vi "getDefaultData.vi"(8 "error in (no error)":errorcluster, 11 "DeviceData in":refnum<class "DeviceData.lvclass">) -> (0 "error out":errorcluster, 1 "calibratedValues":dbl[](array[numeric]), 2 "channelAddresses":string[](array[string]), 3 "DeviceData out":refnum<class "DeviceData.lvclass">)   [LabVIEW 2009, in "DataMappers.lvlib" / "DeviceData.lvclass"]
uses:
  DeviceData.lvclass
  DeviceData.lvclass/DeviceData.ctl
  DatabaseHelpers/Database Objects/ChannelArray/ChannelArray.lvclass
  DatabaseHelpers/Database Objects/device/device.lvclass
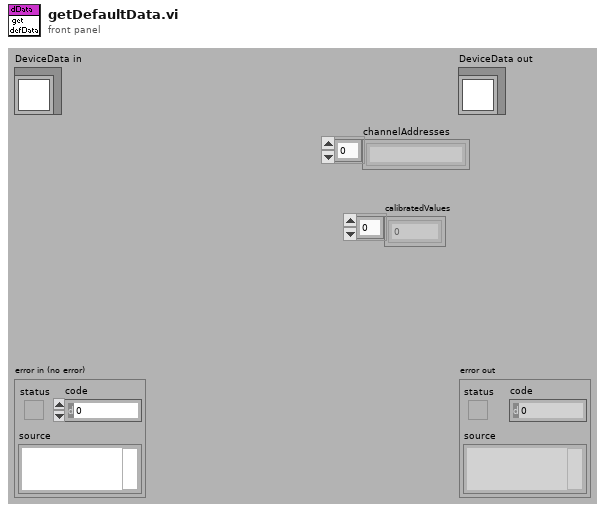
[diagram p1: front panel]
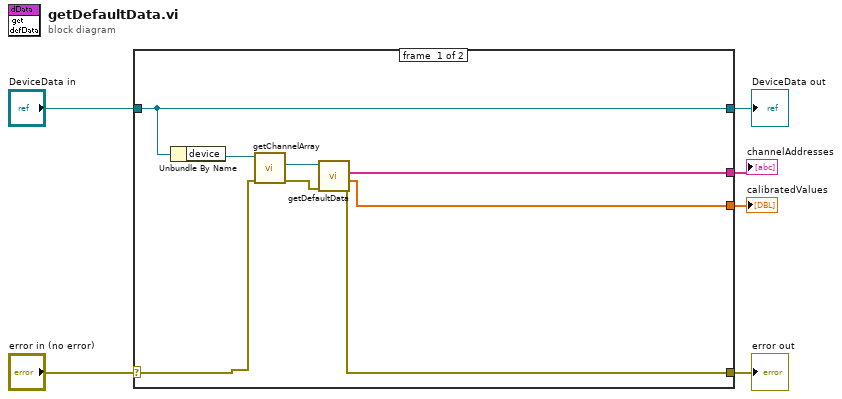
[diagram p0: block diagram]
diagram:
  n1 = case shown="No Error" "error in (no error)" {
    selector: "error in (no error)" -> [w8 w16]
    tunnel: [w7 w16] -> w5
    tunnel: [w14 w15] -> w3
    tunnel: "DeviceData in" -> [w14 w15]
    tunnel: [w10 _] -> w1
    tunnel: [w9 _] -> w2
    frame #0 {
      n2 = Unbundle By Name(w14) -> ("device"=w13:refnum<class "device.lvclass">)
      n3 = call "getChannelArray.vi"("error in (no error)"=w8, "device.lvclass in"=w13) -> ("error out"=w11:errorcluster, "ChannelArray.lvclass"=w12:refnum<class "ChannelArray.lvclass">)  [unwired: 7 in, 1 out]
      n4 = call "getDefaultData.vi"("error in (no error)"=w11, "ChannelArray in"=w12) -> ("error out"=w7:errorcluster, "calibratedValues"=w9:dbl[], "channelAddresses"=w10:string[])  [unwired: 6 in, 1 out]
    }
    frame #1 {
    }
  }
  "error out" <- w5
  "DeviceData out" <- w3
  "calibratedValues" <- w2
  "channelAddresses" <- w1
